vi "Get Mixer.vi"(8 "error in (no error)":errorcluster, 9 "Mix Btn Ref":refnum<vi>, 10 "Speed Ref":refnum<vi>, 11 "data":T1 {"Rotate_IND" items=["стоп", "Качалка Режим Авто", "Качалка Режим Ручной"]; "Termex_IND" items=["Термостат старт"=1, "Термостат стоп"=0]; "Mix_IND" items=["Мешалка движение вперёд"=1, "Мешалка движение назад"=2, "Мешалка стоп"=0]}) -> (0 "error out":errorcluster)   [LabVIEW 2023, in "GUI.lvlib" / "gui.lvclass"]
uses:
  gui.lvclass
  gui.lvclass/gui.ctl
  Modbus PLC/Modbus PLC/Data.ctl
  Modbus PLC/Modbus PLC/Modbus PLC.lvclass
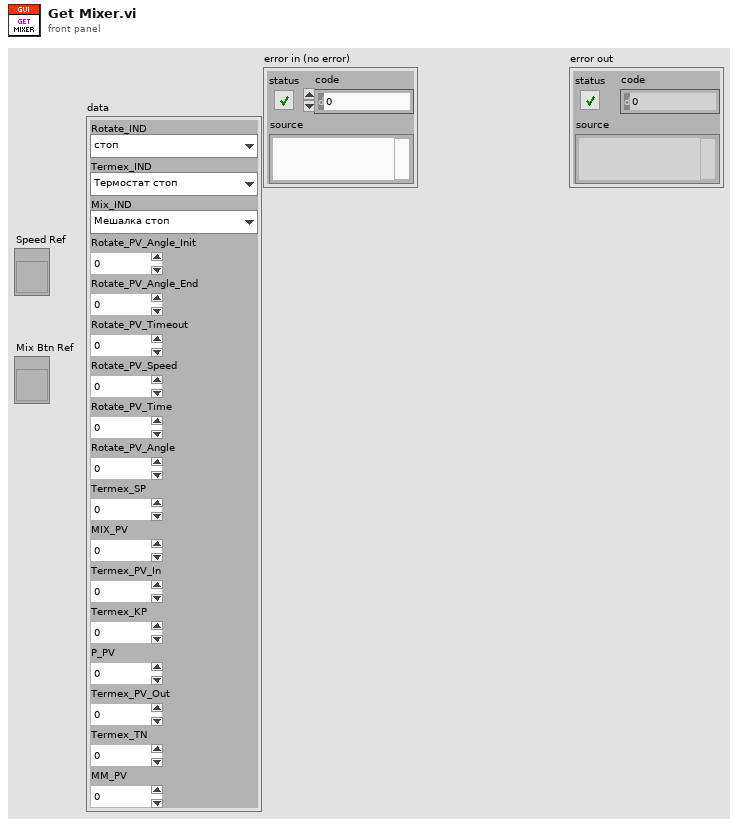
[diagram p1: front panel]
types:
  T1 = typedef "Modbus PLC.lvlib/Modbus PLC.lvclass/Data.ctl" = cluster{"Rotate_IND":u16, "Termex_IND":u16, "Mix_IND":u16, "Rotate_PV_Angle_Init":u16, "Rotate_PV_Angle_End":u16, "Rotate_PV_Timeout":u16, "Rotate_PV_Speed":u16, "Rotate_PV_Time":u16, "Rotate_PV_Angle":u16, "Termex_SP":sgl, "MIX_PV":u16, "Termex_PV_In":sgl, "Termex_KP":sgl, "P_PV":sgl, "Termex_PV_Out":sgl, "Termex_TN":sgl, "MM_PV":sgl}
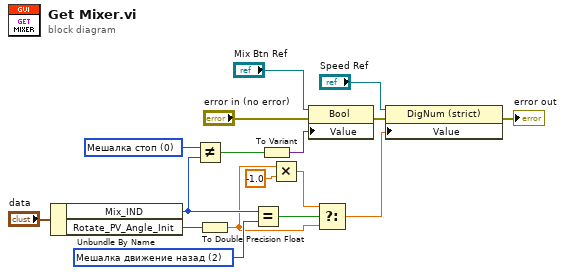
[diagram p0: block diagram]
diagram:
  w11 = u16 2 items=["Мешалка движение вперёд"=1, "Мешалка движение назад"=2, "Мешалка стоп"=0] ("Mix_IND")
  w16 = u16 0 items=["Мешалка движение вперёд"=1, "Мешалка движение назад"=2, "Мешалка стоп"=0] ("Mix_IND")
  n1 = Unbundle By Name("data") -> ("Mix_IND"=w12:u16, "Rotate_PV_Angle_Init"=w8:u16)
  n2 = Not Equal?(x=w16, y=w12) -> (x != y?=w13:bool)
  n3 = To Double Precision Float(number=w8) -> (double precision float=w6:dbl)
  n4 = Equal?(x=w12, y=w11) -> (x = y?=w10:bool)
  n5 = To Variant(anything=w13) -> (Variant=w14:variant)
  n6 = Multiply(x=w6, y=-1.0) -> (x*y=w7:dbl)
  n7 = property class="Bool"(reference="Mix Btn Ref", error in="error in (no error)", "Value"=w14) -> (error out=w3:errorcluster)  [unwired: 1 out]
  n8 = Select(t=w7, s=w10, f=w6) -> (s? t:f=w4:dbl)
  n9 = property class="DigNum (strict)"(reference="Speed Ref", error in=w3, "Value"=w4) -> (error out=→"error out":errorcluster)  [unwired: 1 out]
